vi "add_MultiArrayDimension.vi"(6 "Array":T1, 7 "msg in":string) -> (3 "msg out":string)   [LabVIEW 2015]
uses:
  subs/stringScalar.vi
  subs/u32Scalar.vi
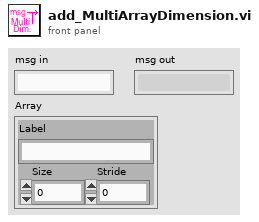
[diagram p1: front panel]
types:
  T1 = cluster{"Label":string, "Size":u32, "Stride":u32}
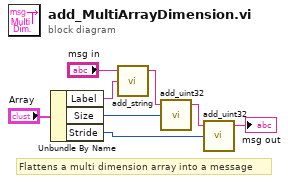
[diagram p0: block diagram]
diagram:
  # "Flattens a multi dimension array into a message"
  n1 = Unbundle By Name("Array") -> ("Label"=w3:string, "Size"=w2:u32, "Stride"=w1:u32)
  n2 = call-poly "add_string.vi"("String"=w3, "msg in"="msg in") -> ("msg out"=w8:string)  [unwired: 3 in]
  n3 = call-poly "add_uint32.vi"("Numeric"=w2, "msg in"=w8) -> ("msg out"=w7:string)  [unwired: 3 in]
  n4 = call-poly "add_uint32.vi"("Numeric"=w1, "msg in"=w7) -> ("msg out"=→"msg out":string)  [unwired: 3 in]
